vi "Read CompactDAQ Settings.vi"(8 "error in (no error)":errorcluster, 11 "CompactDAQ Configuration in":refnum<class "CompactDAQ Configuration.lvclass">) -> (0 "error out":errorcluster, 2 "CompactDAQ Settings":cluster{"Allow Muxing?":bool}, 3 "CompactDAQ Configuration out":refnum<class "CompactDAQ Configuration.lvclass">)   [LabVIEW 2016, in "CompactDAQ Configuration.lvclass"]
uses:
  CompactDAQ Configuration.lvclass
  CompactDAQ Configuration.lvclass/CompactDAQ Configuration.ctl
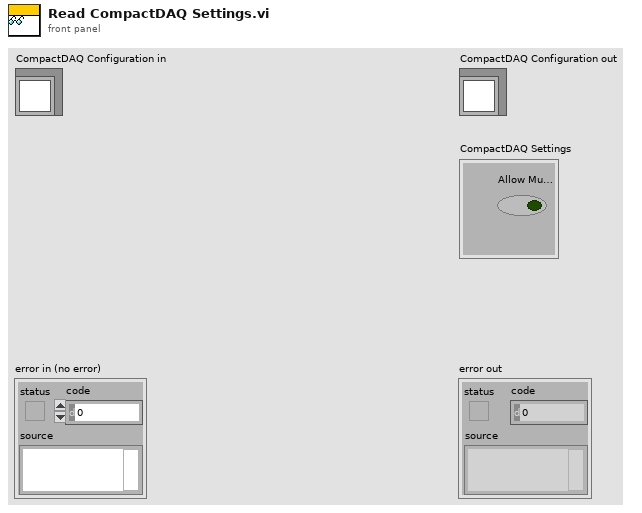
[diagram p1: front panel]
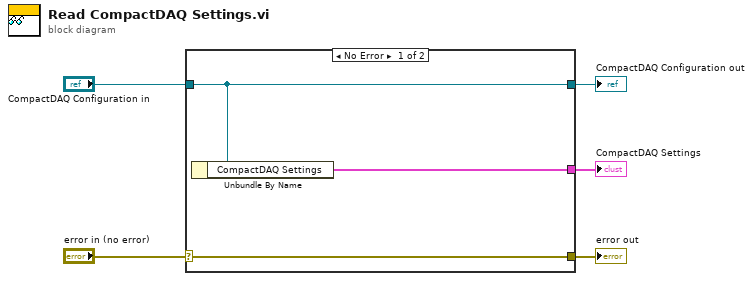
[diagram p0: block diagram]
diagram:
  n1 = case shown="No Error" "error in (no error)" {
    selector: "error in (no error)" -> [w8 w9]
    tunnel: [w8 w9] -> w4
    tunnel: [w7 w10] -> w2
    tunnel: "CompactDAQ Configuration in" -> [w7 w10]
    tunnel: [w6 _] -> w1
    frame No Error {
      n2 = Unbundle By Name(w7) -> ("CompactDAQ Settings"=w6:cluster{"Allow Muxing?":bool})
    }
    frame Error {
    }
  }
  "error out" <- w4
  "CompactDAQ Configuration out" <- w2
  "CompactDAQ Settings" <- w1
